vi "FestoCPX.Station.ButtonLed.Fglb.vi"(7 "Action (get)":T3=enum."get", 8 "error in":errorcluster, 9 "Blink period [ms] (0)":u32, 10 "State":bool, 11 "ButtonLed":T2) -> (0 "error out":errorcluster, 1 "Trigger":bool, 2 "State":T1)   [LabVIEW 2016]
uses:
  FestoCPX.Station.TowerHorn.Fglb.Action.ctl
  FestoCPX.Station.ButtonLed.ctl
  FestoCPX.Station.ButtonsState.ctl
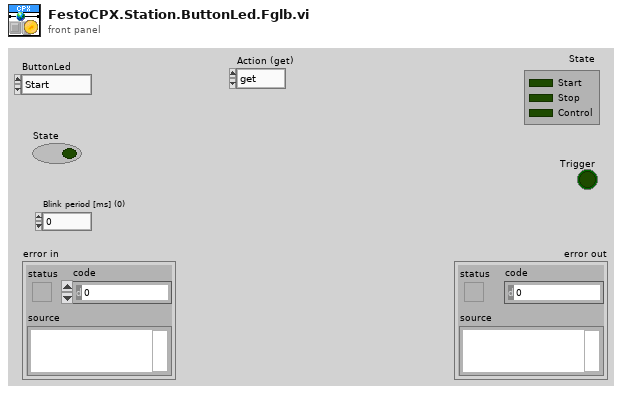
[diagram p1: front panel]
types:
  T1 = typedef "FestoCPX.Station.ButtonsState.ctl" = cluster{"Start":bool, "Stop":bool, "Control":bool}
  T2 = typedef "FestoCPX.Station.ButtonLed.ctl" = enum16{"Start", "Stop", "Control"}
  T3 = typedef "FestoCPX.Station.TowerHorn.Fglb.Action.ctl" = enum16{"init", "set", "get"}
  T4 = cluster{"on":bool, "period":u32, "state":bool, "timer":u32}
  T5 = cluster{"on":bool, "period":u32, "state":bool, "timer":u32}[]
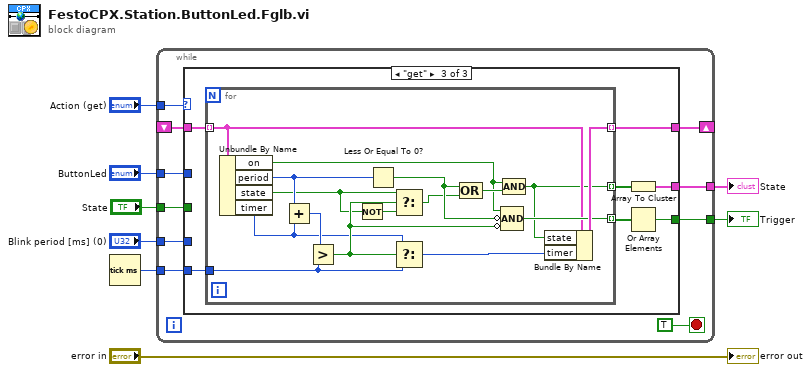
[diagram p0: block diagram]
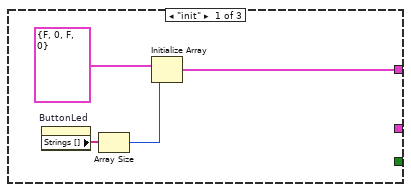
[diagram p2: hidden frame]
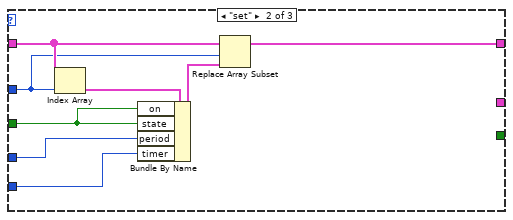
[diagram p3: hidden frame]
diagram:
  n1 = Tick Count (ms)() -> (millisecond timer value=w3:u32)
  n2 = while {
    tunnel: "Action (get)" -> [w17]
    tunnel: "Blink period [ms] (0)" -> [w16]
    tunnel: "ButtonLed" -> [w15]
    shift-right: [w14] -> _
    shift-left: _ -> [w13]
    tunnel: "State" -> [w12]
    tunnel: w3 -> [w11]
    tunnel: [w10] -> w1
    tunnel: [w9] -> w2
    stop <- TRUE stop-if-true
    n3 = case shown="\"get\"" w17 {
      tunnel: w16 -> [_ w27 _]
      tunnel: w15 -> [_ w26 _]
      tunnel: [w19 w30 w35] -> w14
      tunnel: w13 -> [_ w29 w37]
      tunnel: w12 -> [_ w23 _]
      tunnel: w11 -> [_ w24 w36]
      tunnel: [_ _ w31] -> w10
      tunnel: [_ _ w33] -> w9
      frame "init" {
        n4 = property on="ButtonLed" class="Enum (strict)"() -> ("Strings []"=w21:string[])  [unwired: 2 in, 2 out]
        n5 = Array Size(array=w21) -> (size(s)=w20:i32)
        n6 = Initialize Array(T4 {"on"=FALSE, "period"=0, "state"=FALSE, "timer"=0}, w20) -> (w19:T5)
      }
      frame "set" {
        n7 = Index Array(array=w29, index=w26) -> (element=w28:T4)
        n8 = Bundle By Name(cluster=w28, "on"=w23, "state"=w23, "period"=w27, "timer"=w24) -> (w25:T4)
        n9 = Replace Array Subset(array=w29, new element=w25, index=w26) -> (w30:T5)
      }
      frame "get" {
        n10 = for {
          tunnel: w36 -> [w52]
          tunnel: w37 -> [w40] mode=indexing
          tunnel: [w45] -> w35 mode=indexing
          tunnel: [w39] -> w32 mode=indexing
          tunnel: [w41] -> w34 mode=indexing
          n11 = Unbundle By Name(w40) -> ("on"=w38:bool, "period"=w48:u32, "state"=w47:bool, "timer"=w46:u32)
          n12 = Add(x=w48, y=w46) -> (x+y=w53:u32)
          n13 = Greater?(x=w53, y=w52) -> (0:w49:bool)
          n14 = Not(x=w47) -> (.not. x?=w51:bool)
          n15 = Less Or Equal To 0?(x=w48) -> (x <= 0?=w50:bool)
          n16 = Select(t=w47, s=w49, f=w51) -> (s? t:f=w43:bool)
          n17 = Select(t=w46, s=w49, f=w52) -> (s? t:f=w44:u32)
          n18 = Compound Arithmetic op=OR(w50, w43) -> (w42:bool)
          n19 = Compound Arithmetic op=AND(w38, invert w50, invert w49) -> (w41:bool)
          n20 = Compound Arithmetic op=AND(w38, w42) -> (w39:bool)
          n21 = Bundle By Name(cluster=w40, "state"=w39, "timer"=w44) -> (w45:T4)
        }
        n22 = Array To Cluster(array=w32) -> (cluster=w31:cluster{"[0]":bool, "[1]":bool, "[2]":bool})
        n23 = Or Array Elements(Boolean array=w34) -> (logical OR=w33:bool)
      }
    }
  }
  "Trigger" <- w2
  "State" <- w1
  "error out" <- "error in"
